vi "Get Shape.vi"(11 "Snake in":refnum<class "Snake.lvclass">) -> (1 "Color":u32(colorbox), 2 "Coordinates":cluster{"X":i32, "Y":i32}[](array[cluster]), 3 "Snake out":refnum<class "Snake.lvclass">)   [LabVIEW 2020, in "Snake.lvclass"]
uses:
  Snake.lvclass
  Snake.lvclass/Snake.ctl
  Particle.lvclass
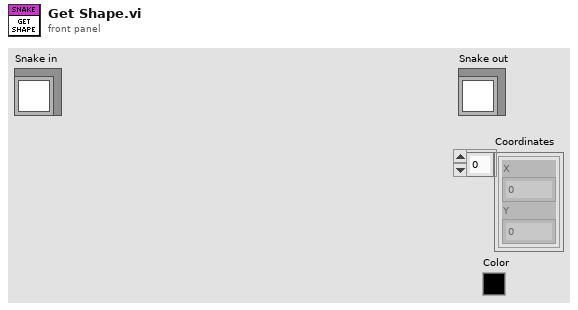
[diagram p1: front panel]
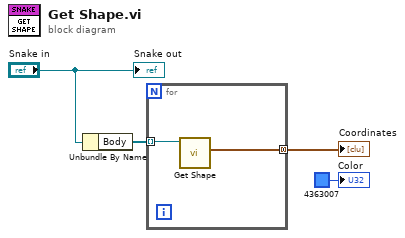
[diagram p0: block diagram]
diagram:
  n1 = Unbundle By Name("Snake in") -> ("Body"=w3:refnum<class "Particle.lvclass">[])
  n2 = for {
    tunnel: w3 -> [w6] mode=indexing
    tunnel: [w5] -> w2 mode=concatenating
    n3 = call-dynamic "Get Shape.vi"("Particle in"=w6) -> ("Coordinates"=w5:cluster{"X":i32, "Y":i32}[])  [unwired: 8 in, 2 out]
  }
  "Coordinates" <- w2
  "Snake out" <- "Snake in"
  "Color" <- u32 4363007 ("Color")
